vi "Initialize.vi"(7 "Serial Configuration":cluster{"Baud Rate":u32}={"Baud Rate"=9600} {"Baud Rate" items=["300"=300, "600"=600, "1200"=1200, "2400"=2400, "4800"=4800, "9600"=9600, "19200"=19200]}, 8 "error in (no error)":errorcluster, 9 "Reset (True)":bool=TRUE, 10 "ID Query (True)":bool=TRUE, 11 "VISA resource name":refnum<visa-resource-name>) -> (0 "error out":errorcluster, 3 "VISA resource name out":refnum<visa-resource-name>)   [LabVIEW 2024, in "BK Precision 8500B Series.lvlib"]
doc: "Establishes communication with the instrument and optionally performs an instrument identification query and/or an instrument reset. It also places the instrument in a default state needed for other instrument driver operations. Therefore, call this VI before calling other instrument driver VIs for this instrument. Generally, you need to call the Initialize VI only once at the beginning of an application."
uses:
  BK Precision 8500B Series.lvlib
panel:
  # "(c) 2019 B&K Precision Corporation.  ALL RIGHTS RESERVED."
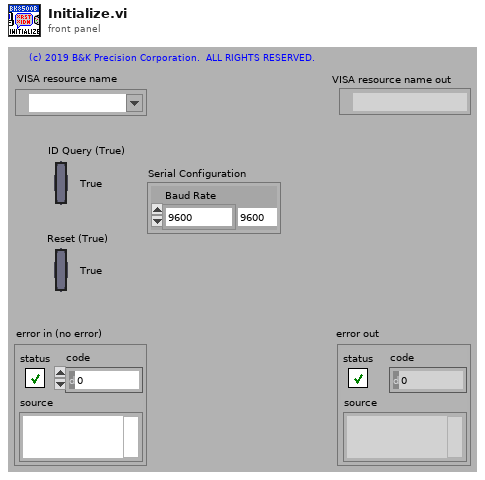
[diagram p1: front panel]
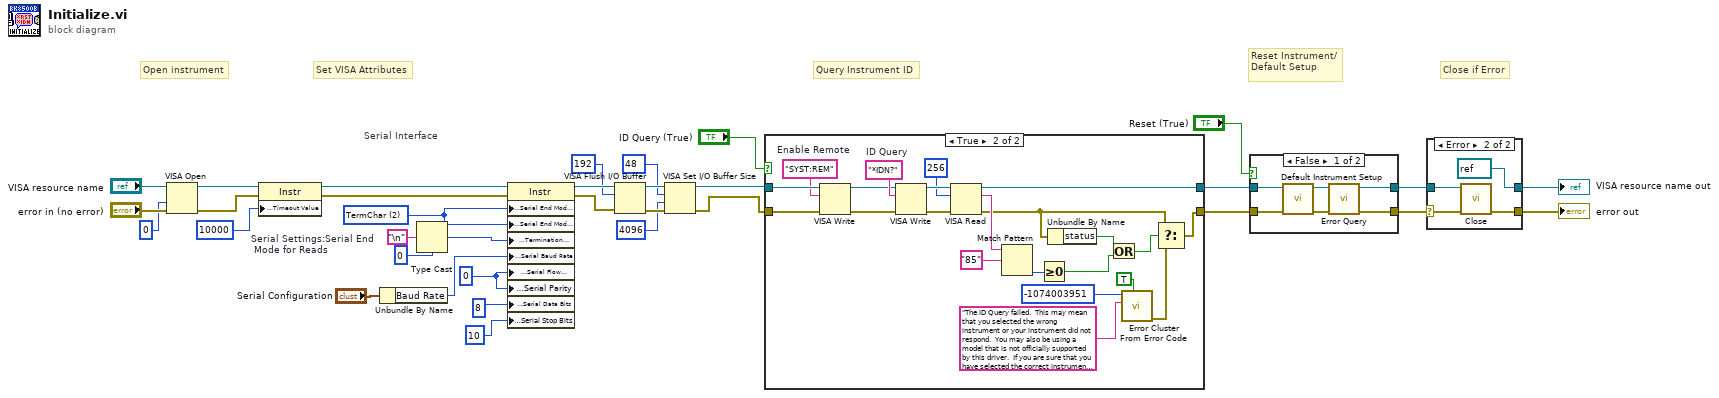
[diagram p0: block diagram]
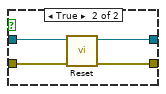
[diagram p3: hidden frame]
diagram:
  w5 = 0
  w7 = u16 2 items=["None", "LastBit", "TermChar"]  # Serial Settings:Serial End  Mode for Reads
  # "Serial Interface"
  # "Set VISA Attributes"
  # "Close if Error"
  # "Query Instrument ID"
  # "Reset Instrument/\nDefault Setup"
  # "Open instrument"
  n1 = VISA Open(access mode=u32 0, error in (no error)="error in (no error)", VISA resource name="VISA resource name") -> (VISA resource name=w18:refnum<visa-resource-name>, error out=w17:errorcluster)  [unwired: 2 in]
  n2 = property class="Instr"(reference=w18, error in=w17, "General Settings:Timeout Value"=u32 10000) -> (reference out=w22:refnum<visa-resource-name>, error out=w21:errorcluster)
  n3 = Unbundle By Name("Serial Configuration") -> ("Baud Rate"=w1:u32)
  n4 = Type Cast(type=u8 0, x="\n" ("Line Feed Constant")) -> (*(type *) &x=w6:u8)
  n5 = property class="Instr"(reference=w22, error in=w21, "Serial Settings:Serial End Mode for Reads"=w7, "Serial Settings:Serial End Mode for Writes"=w7, "Message Based Settings:Termination Character"=w6, "Serial Settings:Serial Baud Rate"=w1, "Serial Settings:Serial Flow Control"=w5, "Serial Settings:Serial Parity"=w5, "Serial Settings:Serial Data Bits"=8, "Serial Settings:Serial Stop Bits"=10) -> (reference out=w13:refnum<visa-resource-name>, error out=w15:errorcluster)
  n6 = VISA Flush I/O Buffer(VISA resource name=w13, mask (16)=u16 192, error in (no error)=w15) -> (VISA resource name out=w16:refnum<visa-resource-name>, error out=w14:errorcluster)
  n7 = VISA Set I/O Buffer Size(VISA resource name=w16, mask (16)=u16 48, size (4096)=u32 4096 ("size (0)"), error in (no error)=w14) -> (VISA resource name out=w20:refnum<visa-resource-name>, error out=w19:errorcluster)
  n8 = case shown="True" "ID Query (True)" {
    tunnel: [w35 w58] -> w33
    tunnel: [w36 w57] -> w34
    tunnel: w20 -> [w36 w38]
    tunnel: w19 -> [w35 w41]
    frame False {
    }
    frame True {
      w37 = "SYST:REM"  # Enable Remote
      w42 = "*IDN?"  # ID Query
      n9 = VISA Write(VISA resource name=w38, write buffer=w37, error in (no error)=w41) -> (VISA resource name out=w39:refnum<visa-resource-name>, error out=w40:errorcluster)  [unwired: 1 out]
      n10 = VISA Write(VISA resource name=w39, write buffer=w42, error in (no error)=w40) -> (VISA resource name out=w55:refnum<visa-resource-name>, error out=w54:errorcluster)  [unwired: 1 out]
      n11 = VISA Read(VISA resource name=w55, byte count=u32 256, error in (no error)=w54) -> (VISA resource name out=w57:refnum<visa-resource-name>, read buffer=w56:string, error out=w46:errorcluster)  [unwired: 1 out]
      n12 = Match Pattern(string=w56, regular expression="85") -> (offset past match=w47:i32)  [unwired: 1 in, 3 out]
      n13 = Greater Or Equal To 0?(x=w47) -> (x >= 0?=w44:bool)
      n14 = Unbundle By Name(w46) -> ("status"=w45:bool)
      n15 = Or(x=w45, y=w44) -> (x .or. y?=w43:bool)
      n16 = call <vilib>:"Error Cluster From Error Code.vi"("show call chain? (False)"=TRUE, "error message (\"\")"="The ID Query failed.  This may mean that you selected the wrong instrument or your instrument did not respond.  You may also be using a model that is not officially supported by this driver.  If you are sure that you have selected the correct instrument and it is responding, try disabling the ID Query." ("Source (VI Name)"), "error code (0)"=-1074003951 ("Code")) -> ("error out"=w51:errorcluster)  [unwired: 6 in]
      n17 = Select(t=w46, s=w43, f=w51) -> (s? t:f=w58:errorcluster)
    }
  }
  n18 = case shown="False" "Reset (True)" {
    tunnel: w33 -> [w63 w65]
    tunnel: [w60 w68] -> w23
    tunnel: w34 -> [w64 w66]
    tunnel: [w61 w67] -> w24
    frame False {
      n19 = call "Default Instrument Setup.vi"("error in (no error)"=w63, "VISA resource name"=w64) -> ("error out"=w59:errorcluster, "VISA resource name out"=w62:refnum<visa-resource-name>)  [unwired: 8 in]
      n20 = call "Error Query.vi"("error in (no error)"=w59, "VISA resource name"=w62) -> ("error out"=w60:errorcluster, "VISA resource name out"=w61:refnum<visa-resource-name>)  [unwired: 6 in, 2 out]
    }
    frame True {
      n21 = call "Reset.vi"("error in (no error)"=w65, "VISA resource name"=w66) -> ("error out"=w68:errorcluster, "VISA resource name out"=w67:refnum<visa-resource-name>)  [unwired: 8 in]
    }
  }
  n22 = case shown="Error" w23 {
    selector: w23 -> [w69 w72]
    tunnel: w24 -> [w70 w73]
    tunnel: [w70 refnum<visa-resource-name> refnum ("VISA resource name out")] -> w26
    tunnel: [w69 w74] -> w25
    frame No Error {
    }
    frame Error {
      n23 = call "Close.vi"("error in (no error)"=w72, "VISA resource name"=w73) -> ("error out"=w74:errorcluster)  [unwired: 9 in]
    }
  }
  "VISA resource name out" <- w26
  "error out" <- w25
